vi "Read OS.vi"() -> ()   [LabVIEW 2020]
panel:
  out "Environment Variable":string
  in  "Envinronment variable":string="USERPROFILE"
  in  "Read env":bool caption="Read"
  in  "Stop Button":bool
  in  "Read":bool
  out "Operating System:Name":string
  out "Operating System:Detailed Name":string
  out "Operating System:Build Number":string
  out "Operating System:Version Number":string
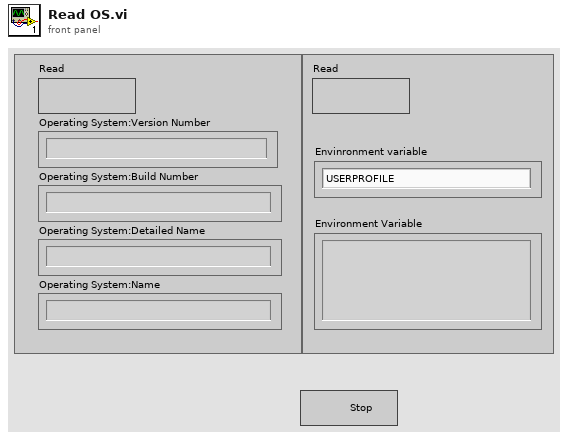
[diagram p1: front panel]
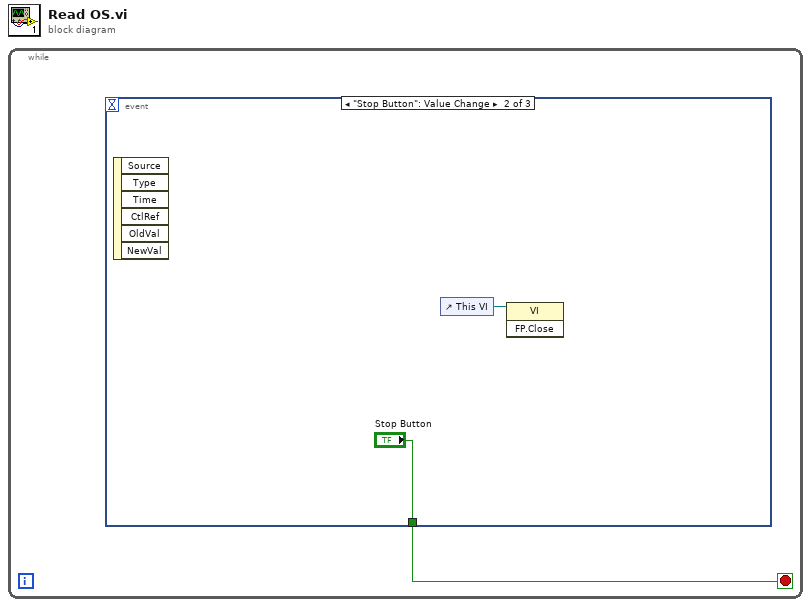
[diagram p0: block diagram]
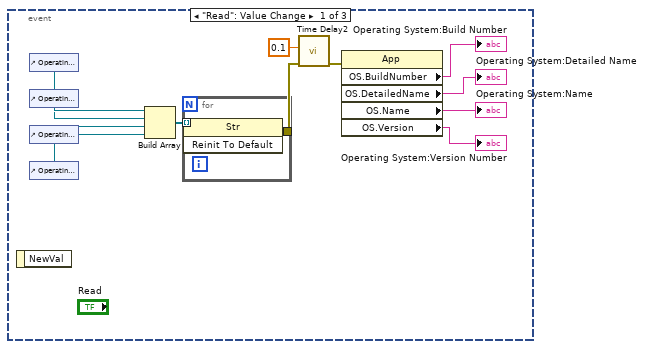
[diagram p2: hidden frame]
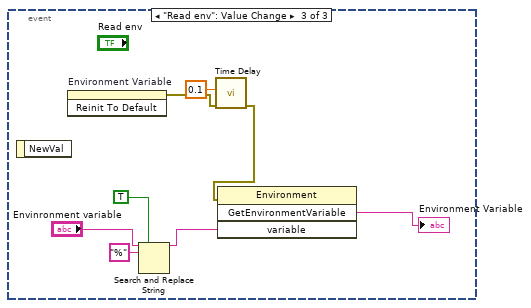
[diagram p3: hidden frame]
diagram:
  n1 = while {
    stop <- w1 stop-if-true
    n2 = event shown="[1] \"Stop Button\": Value Change" {
      selector: _ -> [_ _ _]
      dyn-events: _ -> [_ _ _]
      timeout: _ -> [_ _ _]
      tunnel: [_ "Stop Button" _] -> w1
      event "Read": Value Change {
        n3 = event-data() -> ()  [unwired: 1 in, 1 out]
        n4 = control-ref of="Operating System:Build Number"() -> (w7:refnum<vi>)
        n5 = control-ref of="Operating System:Detailed Name"() -> (w6:refnum<vi>)
        n6 = control-ref of="Operating System:Name"() -> (w5:refnum<vi>)
        n7 = control-ref of="Operating System:Version Number"() -> (w4:refnum<vi>)
        n8 = Build Array(w7, w6, w5, w4) -> (w3:refnum<vi>[])
        n9 = for {
          tunnel: w3 -> [w15] mode=indexing
          tunnel: [w14] -> w2
          n10 = invoke class="Str" method="Reinit To Default"(reference=w15) -> (error out=w14:errorcluster)  [unwired: 2 in, 2 out]
        }
        n11 = call "Time Delay2"("error in (no error)"=w2, "Delay Time (s)"=0.1) -> ("error out"=w9:errorcluster)  [unwired: 9 in]
        n12 = property class="App"(error in=w9) -> ("OS.BuildNumber"=→"Operating System:Build Number":string, "OS.DetailedName"=→"Operating System:Detailed Name":string, "OS.Name"=→"Operating System:Name":string, "OS.Version"=→"Operating System:Version Number":string)  [unwired: 1 in, 2 out]
      }
      event "Stop Button": Value Change {
        n13 = event-data() -> ()  [unwired: 1 in, 6 out]
        n14 = control-ref of="This VI"() -> (w16:refnum<vi>)
        n15 = invoke class="VI" method="FP.Close"(reference=w16) -> ()  [unwired: 2 in, 3 out]
      }
      event "Read env": Value Change {
        n16 = event-data() -> ()  [unwired: 1 in, 1 out]
        n17 = invoke on="Environment Variable" class="Str" method="Reinit To Default"() -> (error out=w20:errorcluster)  [unwired: 3 in, 2 out]
        n18 = Search and Replace String(replace all?=TRUE ("replace all? (F)"), input string="Envinronment variable", search string="%") -> (result string=w22:string)  [unwired: 5 in, 3 out]
        n19 = call "Time Delay"("error in (no error)"=w20, "Delay Time (s)"=0.1) -> ("error out"=w19:errorcluster)  [unwired: 9 in]
        n20 = invoke class="Environment" method="GetEnvironmentVariable"(error in=w19, "variable"=w22) -> ("GetEnvironmentVariable"=→"Environment Variable":string)  [unwired: 2 in, 3 out]
      }
    }
  }
